vi "testFalse.vi"   [LabVIEW 2019, in "AssertionTest.lvlib" / "AssertFalse.lvlib"]
uses:
  AssertFalse.lvlib
  Assertion/Assertion.lvlib
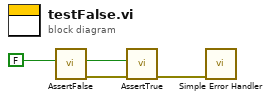
[diagram p0: block diagram]
diagram:
  n1 = call "AssertFalse.vi"("Condition"=FALSE) -> ("error out"=w2:errorcluster, "Result"=w3:bool)  [unwired: 9 in]
  n2 = call "AssertTrue.vi"("error in (no error)"=w2, "Condition"=w3) -> ("error out"=w1:errorcluster)  [unwired: 8 in, 1 out]
  n3 = call <vilib>:"Simple Error Handler.vi"("error in (no error)"=w1) -> ()  [unwired: 4 in, 5 out]
